vi "Cross Process Power No Averaging.vi"(0 "input signal X":waveform(dbl)={"t0"=timestamp(0 s since 1904-01-01), "dt"=1.953125e-05, "Y"=[]}, 1 "input signal Y":waveform(dbl)={"t0"=timestamp(0 s since 1904-01-01), "dt"=1.953125e-05, "Y"=[]}, 2 "window":T2=1 items=["None"=0, "Hanning"=1, "Hamming"=2, "Blackman-Harris"=3, "Exact Blackman"=4, "Blackman"=5, "Flat Top"=6, "4 Term B-Harris "=7, "7 Term B-Harris"=8, "Low Sidelobe"=9, "Force - Exponential"=10, "Blackman Nuttall"=11, "Triangle"=30, "Bartlett-Hanning"=31, "Bohman"=32, "Parzen"=33, "Welch"=34, "Kaiser"=60, "Dolph-Chebyshev"=61, "Gaussian"=62], 3 "force/exp settings":T1={"force window [%]"=50.0, "exponential window [%]"=10.0} {"exponential window [%]" min=0.0 max=100.0 format="%.2f"; "force window [%]" min=0.0 max=100.0 format="%.2f"}, 5 "error in (no error)":errorcluster) -> (14 "complex spectrum":T3={"f0"=0.0, "df"=1.0, "complex spectrum"=[]} {"complex spectrum" format="%.2f"; "df" format="%.2f"; "f0" format="%.2f"}, 19 "error out":errorcluster)   [LabVIEW 2017, in "VibrationAnalysisFunctions.lvlib"]
uses:
  <vilib>/addons/InsightCM/Utilities/Analysis/Vibration/VibrationAnalysisFunctions.lvlib
  <vilib>/addons/_NISVFA/_Shared subVIs/Controls/svc_Window [Dual FFT].ctl
  <vilib>/addons/_NISVFA/_Shared subVIs/Windowing/svfa_Scaled Time Domain Window (1 Ch).vi
  <vilib>/addons/_NISVFA/_Shared subVIs/Windowing/svfa_Scaled Time Domain Window (Array).vi
  <vilib>/Analysis/4window.llb/Force Window.vi
  <vilib>/Analysis/4window.llb/Force Window (DBL).vi
  <vilib>/Analysis/4window.llb/Exponential Window.vi
  <vilib>/Analysis/4window.llb/Exponential Window (DBL).vi
  <vilib>/Utility/error.llb/Error Cluster From Error Code.vi
  <vilib>/Analysis/0measdsp.llb/Scaled Time Domain Window.vi
  <vilib>/Analysis/0measdsp.llb/Scaled Time Domain Window (DBL).vi
  <vilib>/addons/_NISVFA/_Spectrum Processing/subVIs/svfa_Spectrum Info Window to windowTd Type Def.vi
  <vilib>/addons/_NISVFA/_Shared subVIs/Common/svc_Window Parameters.vi
  <vilib>/addons/_NISVFA/_Shared subVIs/Common/svc_Get Window Info.vi
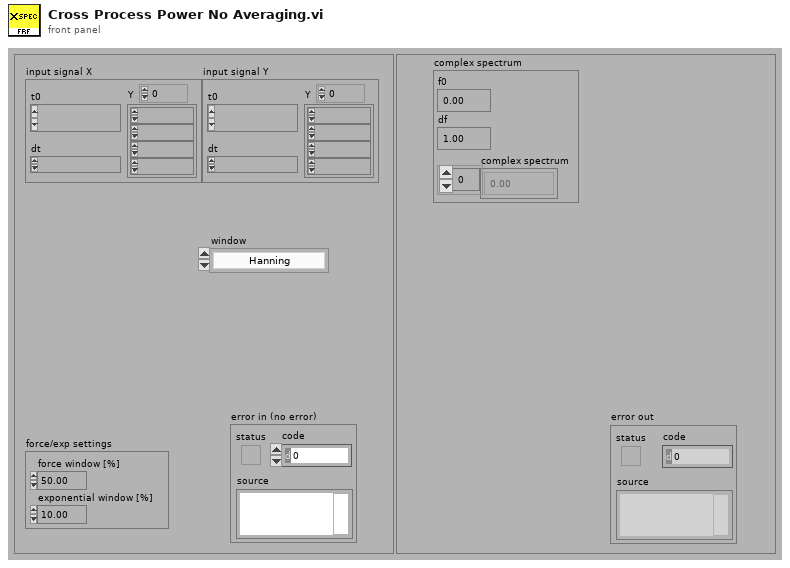
[diagram p1: front panel]
types:
  T1 = cluster{"force window [%]":dbl, "exponential window [%]":dbl}
  T2 = typedef "svc_Window [Dual FFT].ctl" = u32
  T3 = cluster{"f0":dbl, "df":dbl, "complex spectrum":cdb[]}
  T4 = cluster{"df":dbl, "df [Hz]":dbl, "cross spectrum [EUx EUy rms]":cdb[]}
  T5 = typedef "svc_Spectrum Info.ctl" = cluster{"channel name":string, "description":string, "x-axis units":T6, "spectral info":cluster{"spectrum type":T7, "linear/dB":enum16{"linear", "dB"}, "window":u16, "window size":i32, "FFT size":i32}, "engineering units":T8, "custom label":string, "dB reference [EU]":dbl, "peak units":enum16{"rms", "peak", "peak-peak"}, "weighting filter":T9, "spectral density?":bool, "unit label":string, "spectrum skewed?":bool, "complimentary spectrum units":T10}
  T6 = typedef "svc_X-Axis Units.ctl" = u16
  T7 = typedef "svc_Spectrum Type.ctl" = enum16{"FFT Spectrum [complex]", "Amplitude [Magnitude]", "Power [Magnitude^2]", "Cross Spectrum [complex]", "Frequency Response [Complex]"}
  T8 = typedef "svc_Engineering Units Text Ring.ctl" = u16
  T9 = typedef "svc_Weighting Filter Text Ring.ctl" = u16
  T10 = typedef "svc_Complimentary Spectrum Units.ctl" = enum16{"none", "radians", "degrees", "cycles", "imaginary"}
  T11 = cluster{"complex spectrum":cluster{"f0":dbl, "df":dbl, "complex spectrum":cdb[]}, "spectrum info":T5}
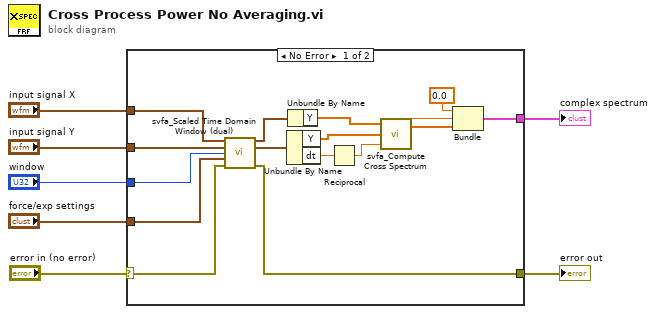
[diagram p0: block diagram]
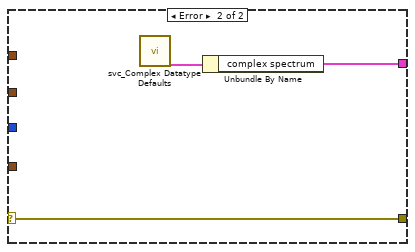
[diagram p2: hidden frame]
diagram:
  n1 = case shown="No Error" "error in (no error)" {
    selector: "error in (no error)" -> [w21 w26]
    tunnel: [w8 w26] -> w7
    tunnel: "input signal X" -> [w23 _]
    tunnel: "input signal Y" -> [w22 _]
    tunnel: [w18 w24] -> w3
    tunnel: "window" -> [w20 _]
    tunnel: "force/exp settings" -> [w19 _]
    frame No Error {
      n2 = call <vilib>:"svfa_Scaled Time Domain Window (dual).vi"("Signal in [X]"=w23, "Signal in [Y]"=w22, "window"=w20, "force/exp settings"=w19, "error in (no error)"=w21) -> ("Windowed signal [X]"=w10:waveform(dbl), "Windowed signal [Y]"=w9:waveform(dbl), "error out"=w8:errorcluster)  [unwired: 4 in, 4 out]
      n3 = Unbundle By Name ("Get Waveform Components")(w9) -> ("Y"=w17:dbl[], "dt"=w16:dbl)
      n4 = Unbundle By Name ("Get Waveform Components")(w10) -> ("Y"=w15:dbl[])
      n5 = Reciprocal(x=w16) -> (1/x=w12:dbl)
      n6 = call <vilib>:"svfa_Compute Cross Spectrum.vi"("sampling frequency [Hz]"=w12, "signal Y [EUy]"=w17, "signal X [EUx]"=w15) -> ("df [Hz]"=w14:dbl, "cross spectrum [EUx EUy rms]"=w11:cdb[])
      n7 = Bundle("df"=0.0, "df [Hz]"=w14, "cross spectrum [EUx EUy rms]"=w11) -> (w18:T4)  [unwired: 1 in]
    }
    frame Error {
      n8 = call <vilib>:"svc_Complex Datatype Defaults.vi"() -> ("complex spectrum"=w25:T11)  [unwired: 11 in, 8 out]
      n9 = Unbundle By Name(w25) -> ("complex spectrum"=w24:T3)
    }
  }
  "error out" <- w7
  "complex spectrum" <- w3
